vi "S_lambda.vi"(6 "Parametry Ziemi":T1={"a - półoś duża"=6378137.0, "b - półoś mała"=6356752.3141999999998} {"b - półoś mała" format="%_20f"; "a - półoś duża" format="%_20g"}, 8 "E":ext format="%#_23g", 9 "fi'[stopnie]":ext format="%#_23g") -> (2 "S_lambda":ext)   [LabVIEW 2012, in "Biblioteka moduł map v3.lvlib" / "Konwersja wsp.lvlib" / "UTM.lvlib" / "Konwersja z UTM na wsp geograficzne.lvlib"]
uses:
  Konwersja z UTM na wsp geograficzne.lvlib
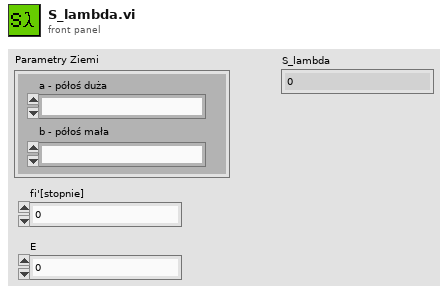
[diagram p1: front panel]
types:
  T1 = cluster{"a - półoś duża":ext, "b - półoś mała":ext}
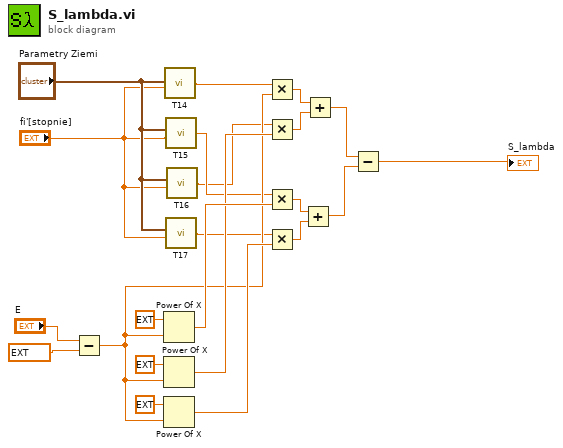
[diagram p0: block diagram]
diagram:
  n1 = Subtract(x="E", y=ext 500000.0 ("FE")) -> (x-y=w10:ext)
  n2 = Power Of X(1:w10, 2:ext 3.0 ("y")) -> (0:w17:ext)
  n3 = Power Of X(1:w10, 2:ext 5.0 ("y")) -> (0:w16:ext)
  n4 = Power Of X(1:w10, 2:ext 7.0 ("y")) -> (0:w15:ext)
  n5 = call "T14.vi"("Parametry Ziemi"="Parametry Ziemi", "fi'"="fi'[stopnie]") -> ("T14"=w6:ext)  [unwired: 6 in]
  n6 = call "T15.vi"("Parametry Ziemi"="Parametry Ziemi", "fi'"="fi'[stopnie]") -> ("T15"=w5:ext)  [unwired: 6 in]
  n7 = call "T17.vi"("Parametry Ziemi"="Parametry Ziemi", "fi'"="fi'[stopnie]") -> ("T17"=w3:ext)  [unwired: 6 in]
  n8 = call "T16.vi"("Parametry Ziemi"="Parametry Ziemi", "fi'"="fi'[stopnie]") -> ("T16"=w4:ext)  [unwired: 6 in]
  n9 = Multiply(x=w6, y=w10) -> (x*y=w12:ext)
  n10 = Multiply(x=w4, y=w16) -> (x*y=w11:ext)
  n11 = Multiply(x=w5, y=w17) -> (x*y=w14:ext)
  n12 = Multiply(x=w3, y=w15) -> (x*y=w13:ext)
  n13 = Add(x=w14, y=w13) -> (x+y=w8:ext)
  n14 = Add(x=w12, y=w11) -> (x+y=w9:ext)
  n15 = Subtract(x=w9, y=w8) -> (x-y=→"S_lambda":ext)
